vi "例程32-均匀白噪声波形VI的使用.vi"() -> ()   [LabVIEW 2016]
uses:
  <vilib>/measure/NI_MABase.lvlib
panel:
  out "波形图":waveform(dbl)(graph)
  out "signal out":waveform(dbl) caption="信号输出"
  out "error out":errorcluster caption="错误输出"
  in  "amplitude":dbl=1.0 caption="幅值" format="%.2p"
  in  "seed":i32=-1 caption="种子"
  in  "error in (no error)":errorcluster caption="错误输入（无错误）"
  in  "reset signal":bool caption="重置信号"
  in  "sampling info":cluster{"Fs":dbl, "#s":dbl}={"Fs"=1000.0, "#s"=1000.0} caption="采样信息" {"Fs" format="%.2p"}
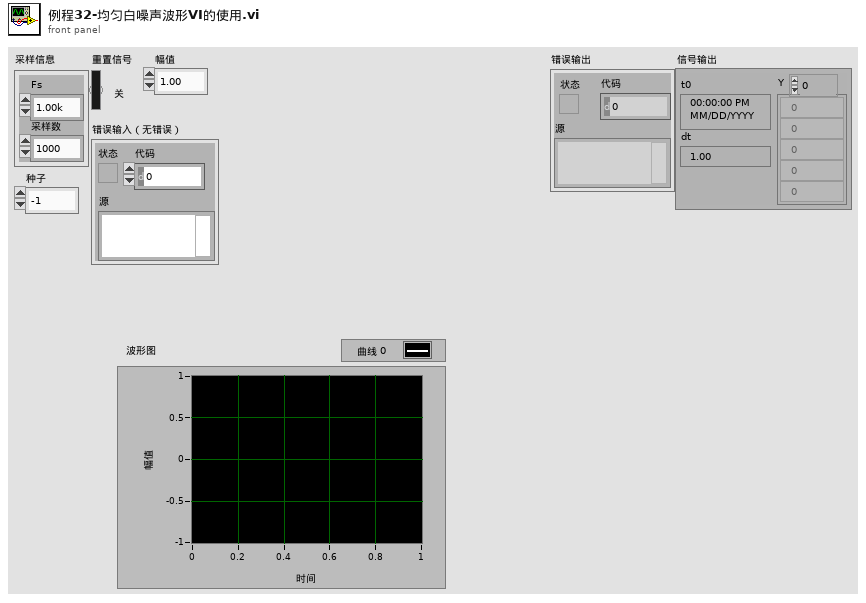
[diagram p1: front panel]
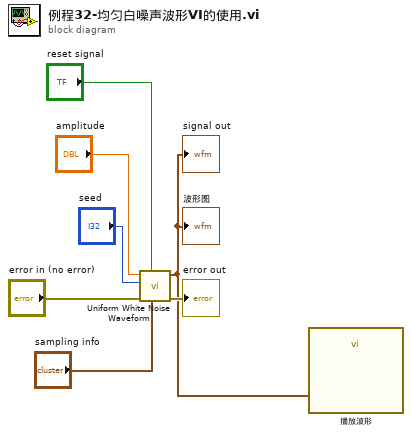
[diagram p0: block diagram]
diagram:
  n1 = call <vilib>:"Uniform White Noise Waveform.vi"("sampling info"="sampling info", "reset signal"="reset signal", "error in (no error)"="error in (no error)", "seed"="seed", "amplitude"="amplitude") -> ("error out"=→"error out":errorcluster, "signal out"=w1:waveform(dbl))  [unwired: 5 in]
  "signal out" <- w1
  "波形图" <- w1
  n2 = call "播放波形"("Data"=w1) -> ()  [unwired: 18 in, 1 out]
